vi "close.vi"(8 "error in (no error)":errorcluster caption="错误输入（无错误）", 11 "DAM0200-Relay 输入":refnum<class "DAM0200-Relay.lvclass">) -> (0 "error out":errorcluster caption="错误输出", 3 "DAM0200-Relay 输出":refnum<class "DAM0200-Relay.lvclass">)   [LabVIEW 2016, in "DAM0200-Relay.lvlib" / "DAM0200-Relay.lvclass"]
uses:
  DAM0200-Relay.lvclass
  DAM0200-Relay.lvclass/DAM0200-Relay.ctl
  <vilib>/Plasmionique/MB Master/MB_Master/MB_Master.lvclass
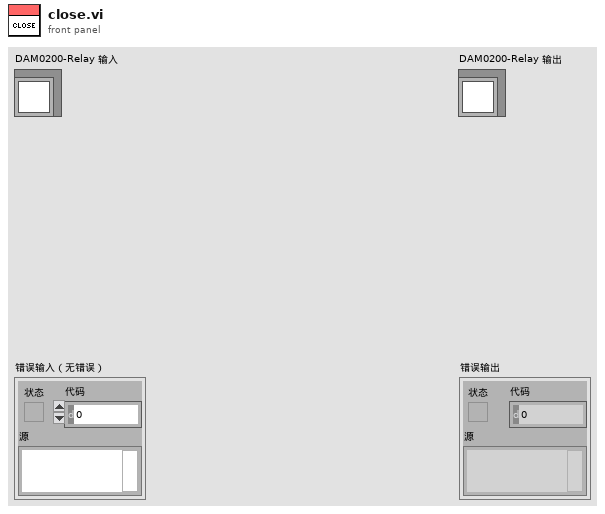
[diagram p1: front panel]
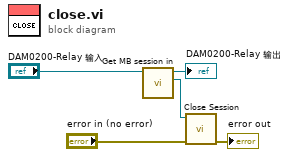
[diagram p0: block diagram]
diagram:
  n1 = call "Get MB session in.vi"("DAM0200-Relay in"="DAM0200-Relay 输入") -> ("MB Serial Master:MB_Master"=w3:refnum<class "MB_Master.lvclass">, "DAM0200-Relay out"=→"DAM0200-Relay 输出":refnum<class "DAM0200-Relay.lvclass">)  [unwired: 9 in]
  n2 = call-dynamic "Close Session.vi"("error in (no error)"="error in (no error)", "MB session in"=w3) -> ("error out"=→"error out":errorcluster)  [unwired: 9 in]
